vi "update named waveforms.vi"(7 "name attribute (NI_ChannelName)":string="NI_ChannelName", 9 "timestamps":timestamp[](array[timestamp]), 10 "values":dbl[](array[numeric]), 11 "names":string[](array[string])) -> (0 "error out":errorcluster, 3 "waveforms out":waveform(dbl)[](array[waveform]))   [LabVIEW 2020]
doc: "Builds and updates waveforms from named signal values sampled at different timestamps for plotting on a waveform chart when different signals are acquired at different rates and/or the sampling rate changes.\n\nBy default, the \"name attribute\" is \"NI_ChannelName\" for consistancy with waveforms produced by DAQmx measurement subVIs.\n\nNote that LabView plots signals that have the same timestamp but varying sampling frequencies in time as expected, but visual glitches appear occasionally when values have different timestamps in the same graph."
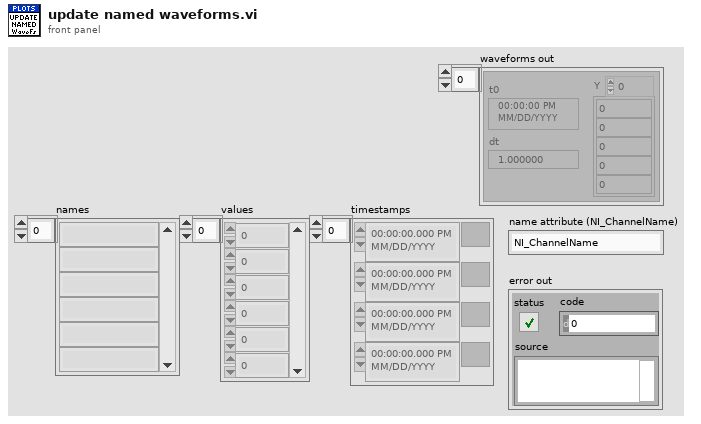
[diagram p1: front panel]
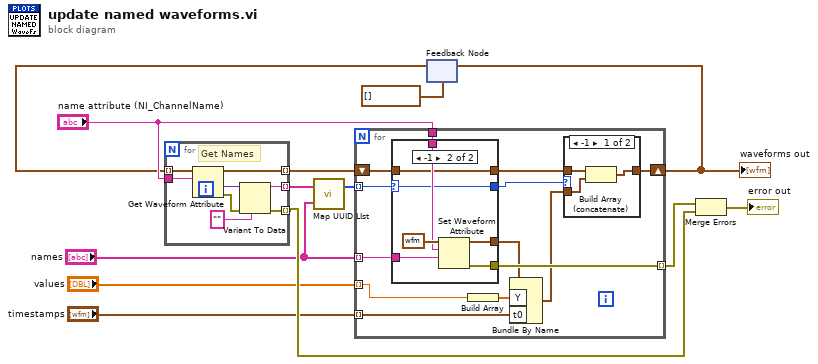
[diagram p0: block diagram]
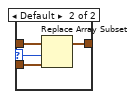
[diagram p2: hidden frame]
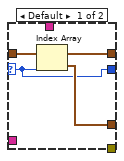
[diagram p3: hidden frame]
diagram:
  n1 = feedback #1(waveform(dbl)[] []) -> (w2:waveform(dbl)[])
  n2 = for {
    tunnel: "name attribute (NI_ChannelName)" -> [w21]
    tunnel: w2 -> [w20] mode=indexing
    tunnel: [w16] -> w5 mode=indexing
    tunnel: [w15] -> w13 mode=indexing
    tunnel: [w14] -> w4 mode=indexing
    # "Get Names"
    n3 = Get Waveform Attribute(6:w21, 7:w20) -> (0:w18:errorcluster, 1:w17:variant, 3:w16:waveform(dbl))  [unwired: 2 in, 1 out]
    n4 = Variant To Data(error in=w18, type="", Variant=w17) -> (data=w14:string, error out=w15:errorcluster)
  }
  n5 = call "Map UUID LIst.vi"("UUIDs"="names", "UUID List"=w4) -> ("indices"=w7:i32[])  [unwired: 1 out]
  n6 = for {
    tunnel: "names" -> [w32] mode=indexing
    tunnel: w7 -> [w34] mode=indexing
    tunnel: "values" -> [w23] mode=indexing
    tunnel: "timestamps" -> [w22] mode=indexing
    tunnel: "name attribute (NI_ChannelName)" -> [w30]
    tunnel: [w29] -> w11 mode=indexing
    shift-right: [w26] -> w3
    shift-left: w5 -> [w33]
    n7 = case shown="-1" w34 {
      selector: w34 -> [w42 w45]
      tunnel: w33 -> [w43 w47]
      tunnel: [w43 w47] -> w27
      tunnel: w32 -> [_ w50]
      tunnel: [_ w49] -> w29
      tunnel: w30 -> [_ w48]
      tunnel: [w44 w46] -> w28
      tunnel: [w42 w45] -> w24
      frame Default {
        n8 = Index Array(array=w43, index=w42) -> (element=w44:waveform(dbl))
      }
      frame -1 {
        n9 = Set Waveform Attribute(5:w50, 6:w48, 7:waveform(dbl) {"t0"=timestamp(0 s since 1904-01-01), "dt"=1.0, "Y"=[]} ("Waveform")) -> (0:w49:errorcluster, 3:w46:waveform(dbl))  [unwired: 1 in, 1 out]
      }
    }
    n10 = Build Array(w23) -> (w31:dbl[])
    n11 = Bundle By Name(cluster=w28, "Y"=w31, "t0"=w22) -> (w25:waveform(dbl))
    n12 = case shown="-1" w24 {
      selector: w24 -> [_ w38]
      tunnel: w27 -> [w37 w41]
      tunnel: [w35 w40] -> w26
      tunnel: w25 -> [w36 w39]
      frame -1 {
        n13 = Build Array (concatenate)(w37, w36) -> (w35:waveform(dbl)[])
      }
      frame Default {
        n14 = Replace Array Subset(array=w41, new element=w39, index=w38) -> (w40:waveform(dbl)[])
      }
    }
  }
  "waveforms out" <- w3
  n15 = feedback-in #1(w3) -> ()
  n16 = Merge Errors(w11, w13) -> (→"error out":errorcluster)
